vi "mxwScript_Cmnd2Str_endGeneration.vi"(8 "error in (no error)":errorcluster, 11 "data":variant) -> (0 "error out":errorcluster, 3 "outputString":string)   [LabVIEW 2020]
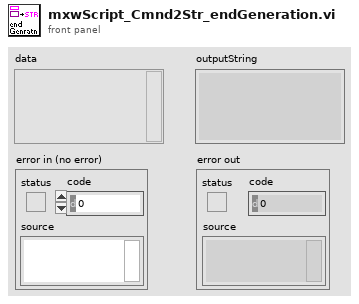
[diagram p1: front panel]
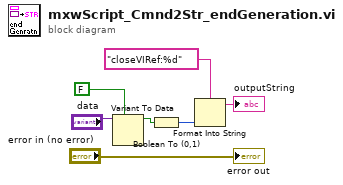
[diagram p0: block diagram]
diagram:
  n1 = Variant To Data(type=FALSE, Variant="data") -> (data=w2:bool)  [unwired: 1 in, 1 out]
  n2 = Boolean To (0,1)(Boolean=w2) -> (0, 1=w1:i16)
  n3 = Format Into String(format string="closeVIRef:%d", w1) -> (resulting string=→"outputString":string)  [unwired: 2 in, 1 out]
  "error out" <- "error in (no error)"
